vi "Aim Robot - old.vi"(10 "Drive Speed":dbl, 11 "RobotDriveDevRef":T1={"DevStatus"={"status"=FALSE, "code"=0, "source"=""}, "Motors[]"=[], "Square Inputs"=FALSE, "Max Output"=1.0}) -> (0 "Error Out":string, 3 "RobotDriveDevRef Out":T1={"DevStatus"={"status"=FALSE, "code"=0, "source"=""}, "Motors[]"=[], "Square Inputs"=FALSE, "Max Output"=1.0})   [LabVIEW 2016]
uses:
  <vilib>/Rock Robotics/WPI/RobotDrive/WPI_RobotDriveDevRef.ctl
  <vilib>/Rock Robotics/WPI/MotorControl/WPI_MotorControlDeviceRef.ctl
  <vilib>/Rock Robotics/WPI/MotorControl/WPI_MotorControlType.ctl
  <vilib>/Rock Robotics/SystemInterfaces/DIO/FPGA_DIOPWMChannel.ctl
  <vilib>/Rock Robotics/WPI/PWM/WPI_PWMDeadband.ctl
  <vilib>/Rock Robotics/WPI/Relay/WPI_RelayValue.ctl
  <vilib>/Rock Robotics/Network Tables/NT Read Boolean.vi
  <vilib>/Rock Robotics/WPI/RobotDrive/WPI_RobotDriveArcadeDrive_Standard(NoSaturation).vi
  <vilib>/Rock Robotics/Network Tables/NT Write Numeric Array.vi
  <vilib>/Rock Robotics/Network Tables/NT Read Number.vi
  Robot Global Data.vi
panel:
  out "Drive Motor Values":dbl[](array[numeric])
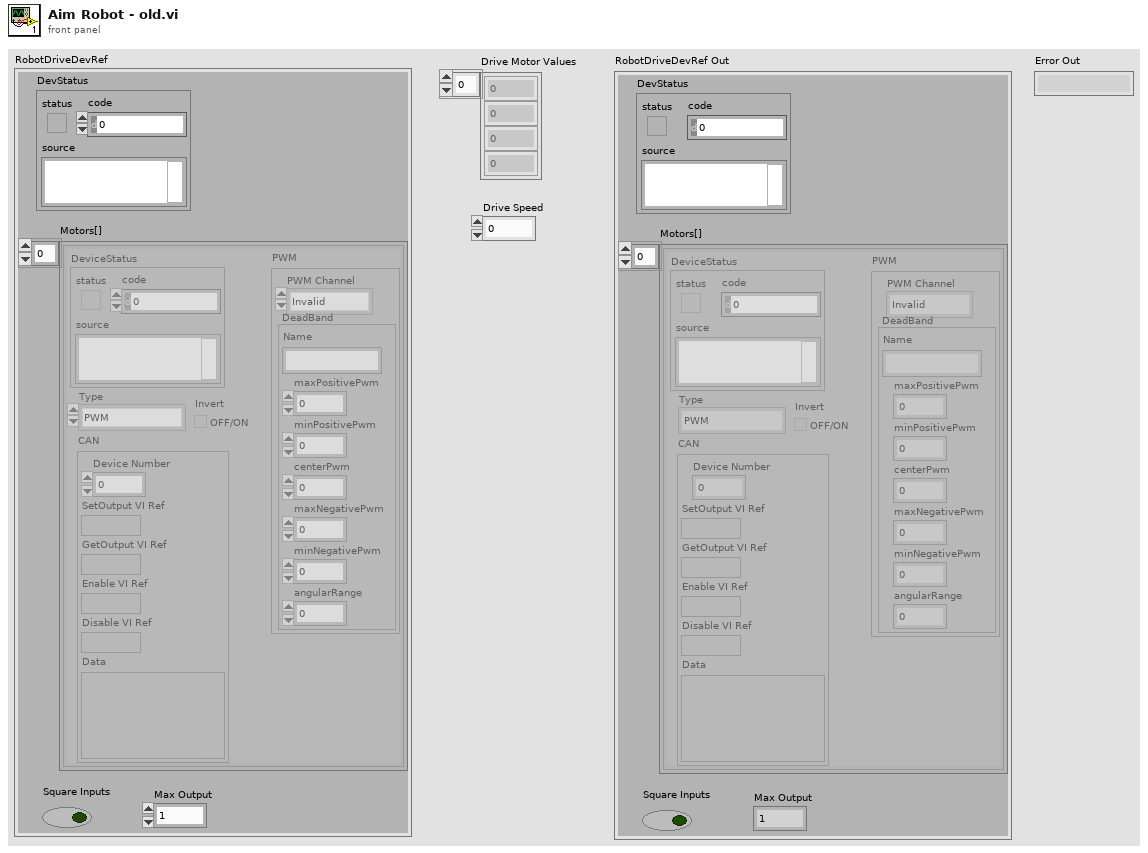
[diagram p1: front panel]
types:
  T1 = typedef "WPI_RobotDriveDevRef.ctl" = cluster{"DevStatus":errorcluster, "Motors[]":T2[], "Square Inputs":bool, "Max Output":dbl}
  T2 = typedef "WPI_MotorControlDeviceRef.ctl" = cluster{"DeviceStatus":errorcluster, "Type":T3, "PWM":cluster{"PWM Channel":T4, "DeadBand":T5}, "CAN":cluster{"Device Number":u8, "SetOutput VI Ref":variant, "GetOutput VI Ref":variant, "Enable VI Ref":variant, "Disable VI Ref":variant, "Data":variant}, "Invert":bool}
  T3 = typedef "WPI_MotorControlType.ctl" = enum16{"PWM", "CAN"}
  T4 = typedef "FPGA_DIOPWMChannel.ctl" = enum8{"PWM 0", "PWM 1", "PWM 2", "PWM 3", "PWM 4", "PWM 5", "PWM 6", "PWM 7", "PWM 8", "PWM 9", "PWM MXP 0", "PWM MXP 1", "PWM MXP 2", "PWM MXP 3", "PWM MXP 4", "PWM MXP 5", "PWM MXP 6", "PWM MXP 7", "PWM MXP 8", "PWM MXP 9", "Invalid"}
  T5 = typedef "WPI_PWMDeadband.ctl" = cluster{"Name":string, "maxPositivePwm":i32, "minPositivePwm":i32, "centerPwm":i32, "maxNegativePwm":i32, "minNegativePwm":i32, "angularRange":u16}
  T6 = typedef "WPI_RelayValue.ctl" = enum16{"Off", "On", "Forward", "Reverse"}
  T7 = typedef "WPI_RelayDevRef.ctl" = cluster{"DevStatus":errorcluster, "Relay Channel":T8, "Relay Direction":T9}
  T8 = typedef "FPGA_DIORelayChannel.ctl" = enum8{"Relay 0", "Relay 1", "Relay 2", "Relay 3", "Invalid"}
  T9 = typedef "WPI_RelayDirection.ctl" = enum16{"Both directions", "Forward only", "Reverse only"}
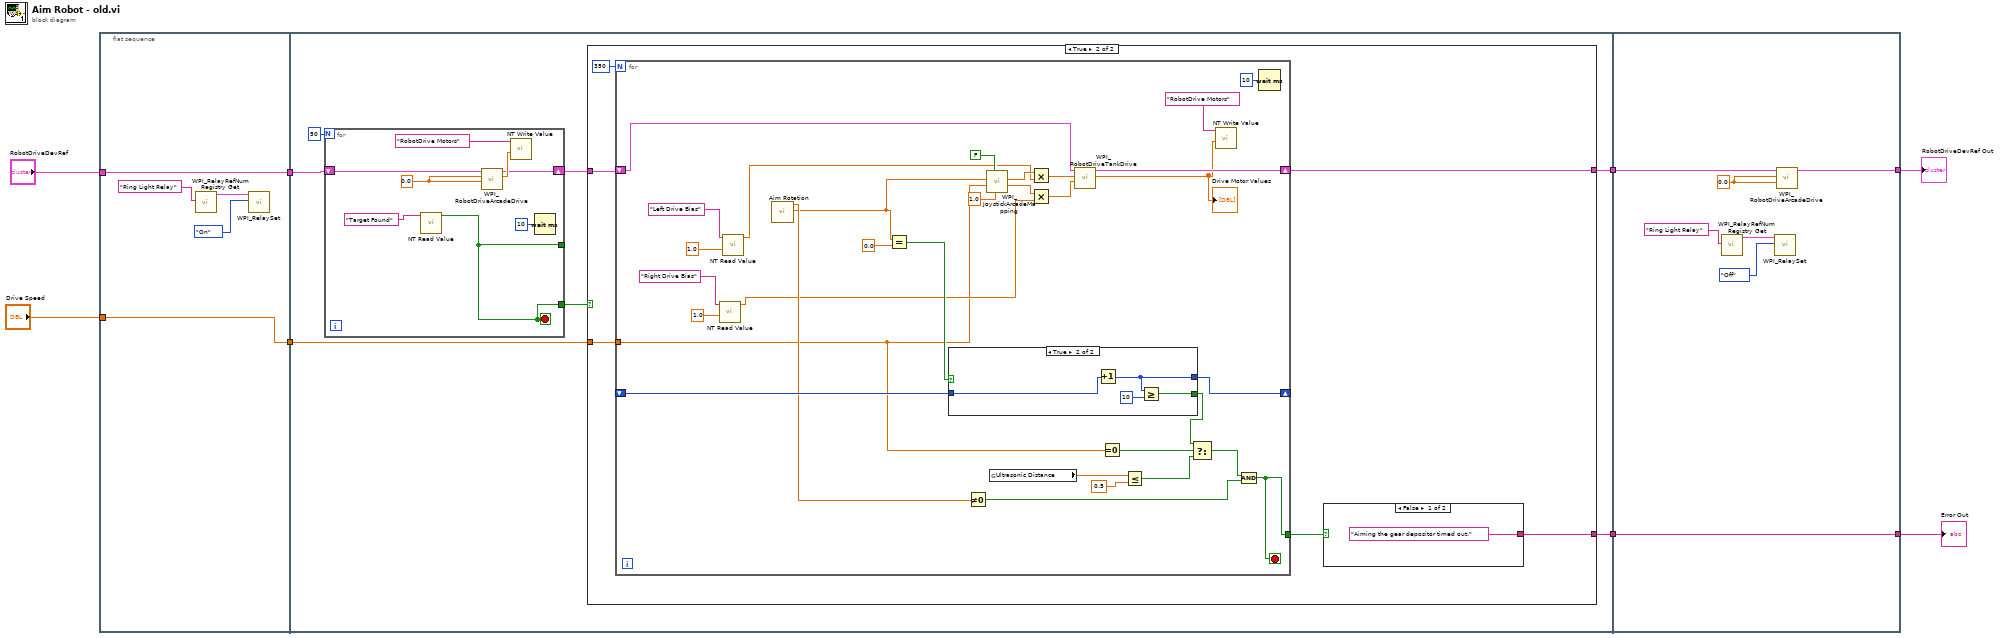
[diagram p0: block diagram]
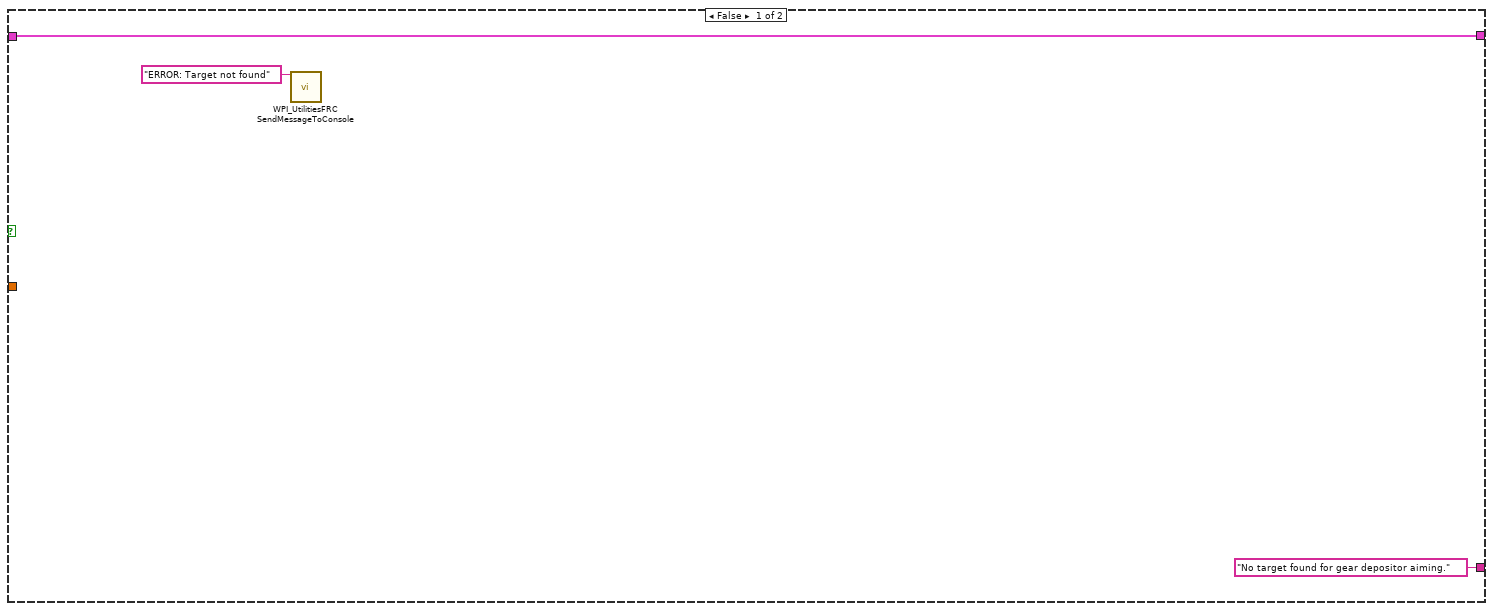
[diagram p2: hidden frame]
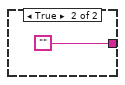
[diagram p3: hidden frame]
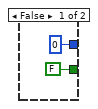
[diagram p4: hidden frame]
diagram:
  n1 = flat-sequence {
    tunnel: [w10] -> w8
    tunnel: "RobotDriveDevRef" -> [w10]
    tunnel: [w9] -> w6
    tunnel: "Drive Speed" -> [w9]
    tunnel: w8 -> [w17]
    tunnel: w6 -> [w16]
    tunnel: [w15] -> w4
    tunnel: [w14] -> w2
    tunnel: w4 -> [w81]
    tunnel: [w79] -> w3
    tunnel: w2 -> [w78]
    tunnel: [w78] -> w1
    frame #0 {
      n2 = call <vilib>:"WPI_RelayRefNum Registry Get.vi"("refnum name"="Ring Light Relay") -> ("RelayDevRef"=w12:T7)  [unwired: 9 in, 1 out]
      n3 = call <vilib>:"WPI_RelaySet.vi"("RelayValue"=WPI_RelayValue."On", "RelayDevRef"=w12) -> ()  [unwired: 8 in, 2 out]
    }
    frame #1 {
      n4 = for {
        N: 50 -> [_]
        tunnel: [w71] -> _
        shift-right: [w72] -> w19
        shift-left: w17 -> [w73]
        tunnel: [w71] -> w18
        stop <- w71 stop-if-true
        w70 = 0.0
        n5 = call-poly <vilib>:"NT Read Value.vi"("Name"="Target Found") -> ("Boolean"=w71:bool)  [unwired: 9 in, 1 out]
        n6 = call-poly <vilib>:"WPI_RobotDriveArcadeDrive.vi"("Y axis value"=w70, "X axis value"=w70, "RobotDriveDevRef"=w73) -> ("Motor Values"=w75:dbl[], "RobotDriveDevRef"=w72:T1)  [unwired: 6 in, 1 out]
        n7 = call-poly <vilib>:"NT Write Value.vi"("Numeric Array"=w75, "Name"="RobotDrive Motors") -> ()  [unwired: 9 in, 1 out]
        n8 = Wait (ms)(milliseconds to wait=u32 10) -> ()  [unwired: 1 out]
      }
      n9 = case shown="True" w18 {
        tunnel: w19 -> [w22 w28]
        tunnel: w16 -> [_ w27]
        tunnel: [w22 w26] -> w15
        tunnel: ["No target found for gear depositor aiming." w24] -> w14
        frame False {
          n10 = call <vilib>:"WPI_UtilitiesFRC SendMessageToConsole.vi"("Message"="ERROR: Target not found") -> ()  [unwired: 14 in, 1 out]
        }
        frame True {
          n11 = for {
            N: 350 -> [_]
            shift-right: [w43] -> w26
            shift-left: w28 -> [w44]
            shift-right: [w60] -> _
            shift-left: _ -> [w61]
            tunnel: w27 -> [w41]
            tunnel: [w38] -> w25
            stop <- w38 stop-if-true
            n12 = call-poly <vilib>:"NT Read Value.vi"("Default Value"=1.0, "Name"="Right Drive Bias") -> ("Numeric"=w47:dbl)  [unwired: 8 in, 1 out]
            n13 = call-poly <vilib>:"NT Read Value.vi"("Default Value"=1.0, "Name"="Left Drive Bias") -> ("Numeric"=w48:dbl)  [unwired: 8 in, 1 out]
            n14 = call "Aim Rotation.vi"() -> ("Rotation"=w51:dbl, "Image Size X"=w57:dbl)  [unwired: 10 in]
            n15 = Equal?(x=w51, y=0.0) -> (x = y?=w58:bool)
            n16 = case shown="True" w58 {
              tunnel: [0 w68] -> w60
              tunnel: w61 -> [_ w69]
              tunnel: [FALSE w66] -> w36
              frame False {
              }
              frame True {
                n17 = Increment(x=w69) -> (x+1=w68:i32)
                n18 = Greater Or Equal?(x=w68, y=10) -> (x >= y?=w66:bool)
              }
            }
            n19 = Not Equal To 0?(x=w57) -> (x != 0?=w56:bool)
            n20 = call <vilib>:"WPI_JoystickArcadeMapping.vi"("Max Output"=1.0, "Square Inputs"=FALSE, "Y axis value"=w41, "X axis value"=w51) -> ("Right Motor Value"=w50:dbl, "Left Motor Value"=w49:dbl)  [unwired: 6 in]
            n21 = global read "Robot Global Data.vi" "Ultrasonic Distance"() -> (w35:dbl)
            n22 = Multiply(x=w49, y=w48) -> (x*y=w46:dbl)
            n23 = Multiply(x=w50, y=w47) -> (x*y=w45:dbl)
            n24 = call <vilib>:"WPI_RobotDriveTankDrive.vi"("Right axis value"=w45, "Left axis value"=w46, "RobotDriveDevRef"=w44) -> ("Motor Values"=w42:dbl[], "RobotDriveDevRef"=w43:T1)  [unwired: 6 in, 1 out]
            "Drive Motor Values" <- w42
            n25 = Equal To 0?(x=w41) -> (x = 0?=w37:bool)
            n26 = Less Or Equal?(x=w35, y=0.5) -> (x <= y?=w33:bool)
            n27 = Select(t=w36, s=w37, f=w33) -> (s? t:f=w32:bool)
            n28 = call-poly <vilib>:"NT Write Value.vi"("Numeric Array"=w42, "Name"="RobotDrive Motors") -> ()  [unwired: 9 in, 1 out]
            n29 = Compound Arithmetic op=AND(w32, w56) -> (w38:bool)
            n30 = Wait (ms)(milliseconds to wait=u32 10) -> ()  [unwired: 1 out]
          }
          n31 = case shown="False" w25 {
            tunnel: ["Aiming the gear depositor timed out." ""] -> w24
            frame False {
            }
            frame True {
            }
          }
        }
      }
    }
    frame #2 {
      w80 = 0.0 ("X axis value")
      n32 = call <vilib>:"WPI_RelayRefNum Registry Get.vi"("refnum name"="Ring Light Relay") -> ("RelayDevRef"=w83:T7)  [unwired: 9 in, 1 out]
      n33 = call <vilib>:"WPI_RelaySet.vi"("RelayValue"=WPI_RelayValue."Off", "RelayDevRef"=w83) -> ()  [unwired: 8 in, 2 out]
      n34 = call-poly <vilib>:"WPI_RobotDriveArcadeDrive.vi"("Y axis value"=w80, "X axis value"=w80, "RobotDriveDevRef"=w81) -> ("RobotDriveDevRef"=w79:T1)  [unwired: 6 in, 2 out]
    }
  }
  "RobotDriveDevRef Out" <- w3
  "Error Out" <- w1
